vi "Init Rx Data.vi"(7 "Data Access in":refnum<class "Data Access Engine.lvclass">, 8 "error in (no error)":errorcluster, 11 "Parameters":variant) -> (0 "error out":errorcluster, 3 "Rx Loop Data":T1, 5 "Data Access out":refnum<class "Data Access Engine.lvclass">)   [LabVIEW 2016, in "UDP-Custom-Device Engine.lvlib"]
uses:
  UDP-Custom-Device Engine.lvlib
  Rx Loop Data.ctl
  <vilib>/NI/NIVS Inline Async API/_Data Access Engine/Data Access Engine/Types/Write.DVR.ctl
  <vilib>/NI/NIVS Inline Async API/_Data Access Engine/Access Type Classes/Write/Write.lvclass
  <vilib>/NI/NIVS Inline Async API/_Data Access Engine/Data Access Engine/Data Access Engine.lvclass
  Shared/Rx.PacketInfo.ctl
  <vilib>/NI/NIVS Inline Async API/_Data Access Engine/Data Access Engine/Methods/Write.Lookup.vi
  Shared/UDP-Custom-Device Shared.lvlib
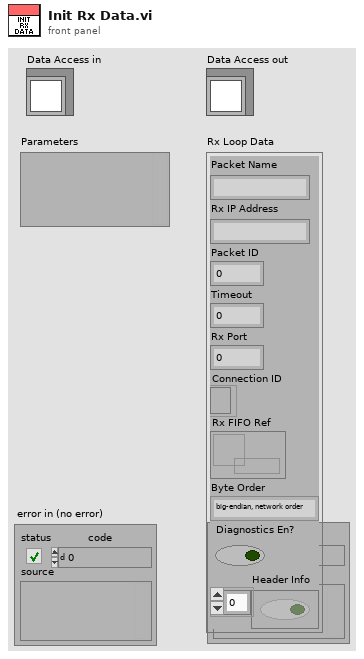
[diagram p1: front panel]
types:
  T1 = typedef "UDP-Custom-Device Engine.lvlib/Rx Loop Data.ctl" = cluster{"Packet Name":string, "Rx IP Address":string, "Packet ID":i32, "Timeout":i32, "Rx Port":i32, "Connection ID":refnum<k16>, "Rx FIFO Ref":T2, "Byte Order":enum16{"big-endian, network order", "native, host order", "little-endian"}, "Diagnostics En?":bool, "Header Info":bool[]}
  T2 = typedef "Data Access Engine.lvlib/Data Access Engine.lvclass/Write.DVR.ctl" = refnum<data-value>
  T3 = typedef "UDP-Custom-Device Shared.lvlib/Rx.PacketInfo.ctl" = cluster{"Packet Name":string, "Packet ID":i32, "Timeout":i32, "Rx IP Address":string, "Rx Port":i32, "Endianness":u16, "Diagnostics En?":bool, "Header Info":bool[]}
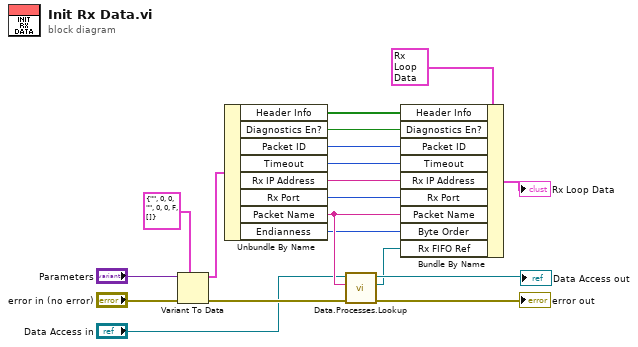
[diagram p0: block diagram]
diagram:
  n1 = Variant To Data(error in="error in (no error)", type=T3 {"Packet Name"="", "Packet ID"=0, "Timeout"=0, "Rx IP Address"="", "Rx Port"=0, "Endianness"=0, "Diagnostics En?"=FALSE, "Header Info"=[]} ("Packet Info"), Variant="Parameters") -> (data=w16:T3, error out=w9:errorcluster)
  n2 = Unbundle By Name(w16) -> ("Header Info"=w1:bool[], "Diagnostics En?"=w2:bool, "Packet ID"=w10:i32, "Timeout"=w11:i32, "Rx IP Address"=w12:string, "Rx Port"=w13:i32, "Packet Name"=w8:string, "Endianness"=w3:u16)
  n3 = call-poly <vilib>:"Data.Processes.Lookup.vi"("error in (no error)"=w9, "Name"=w8, "Data Access API in"="Data Access in") -> ("error out"=→"error out":errorcluster, "Ref"=w4:T2, "Data Access API out"=→"Data Access out":refnum<class "Data Access Engine.lvclass">)  [unwired: 5 in, 1 out]
  n4 = Bundle By Name(cluster=T1 {"Packet Name"="", "Rx IP Address"="", "Packet ID"=0, "Timeout"=0, "Rx Port"=0, "Connection ID"=refnum, "Rx FIFO Ref"=refnum, "Byte Order"=enum."big-endian, network order", "Diagnostics En?"=FALSE, "Header Info"=[]} ("Rx Loop Data"), "Header Info"=w1, "Diagnostics En?"=w2, "Packet ID"=w10, "Timeout"=w11, "Rx IP Address"=w12, "Rx Port"=w13, "Packet Name"=w8, "Byte Order"=w3, "Rx FIFO Ref"=w4) -> (→"Rx Loop Data":T1)
